vi "SimpleMotorFF_MinAchieveVel.vi"(9 "Acceleration":dbl, 10 "MaxVoltage":dbl, 11 "SIMPLE_MOTOR_FF":T1 {"Ka" format="%13.4f"; "Kv" format="%13.4f"; "Ks" format="%13.4f"}) -> (3 "MinVelocity":dbl)   [LabVIEW 2019, in "Trajectory_Library.lvlib"]
doc: "Calculates the minimum achievable velocity given a maximum voltage supply and an acceleration. Useful for ensuring that velocity and acceleration constraints for a trapezoidal profile are simultaneously achievable - enter the acceleration constraint, and this will give you a simultaneously-achievable velocity constraint.\n\nParameters:\n - Simple_Motor_FF - Data structure containing constants\n - maxVoltage -The maximum voltage that can be supplied to the motor.\n - Acceleration - The acceleration of the motor.\n\nReturns:\n - MinVelocity - The minimum possible velocity at the given acceleration."
uses:
  Trajectory_Library.lvlib
  TypeDef/SIMPLE_MOTOR_FF.ctl
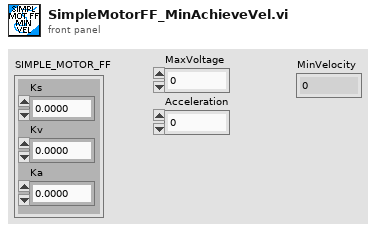
[diagram p1: front panel]
types:
  T1 = typedef "Trajectory_Library.lvlib/SIMPLE_MOTOR_FF.ctl" = cluster{"Ks":dbl, "Kv":dbl, "Ka":dbl}
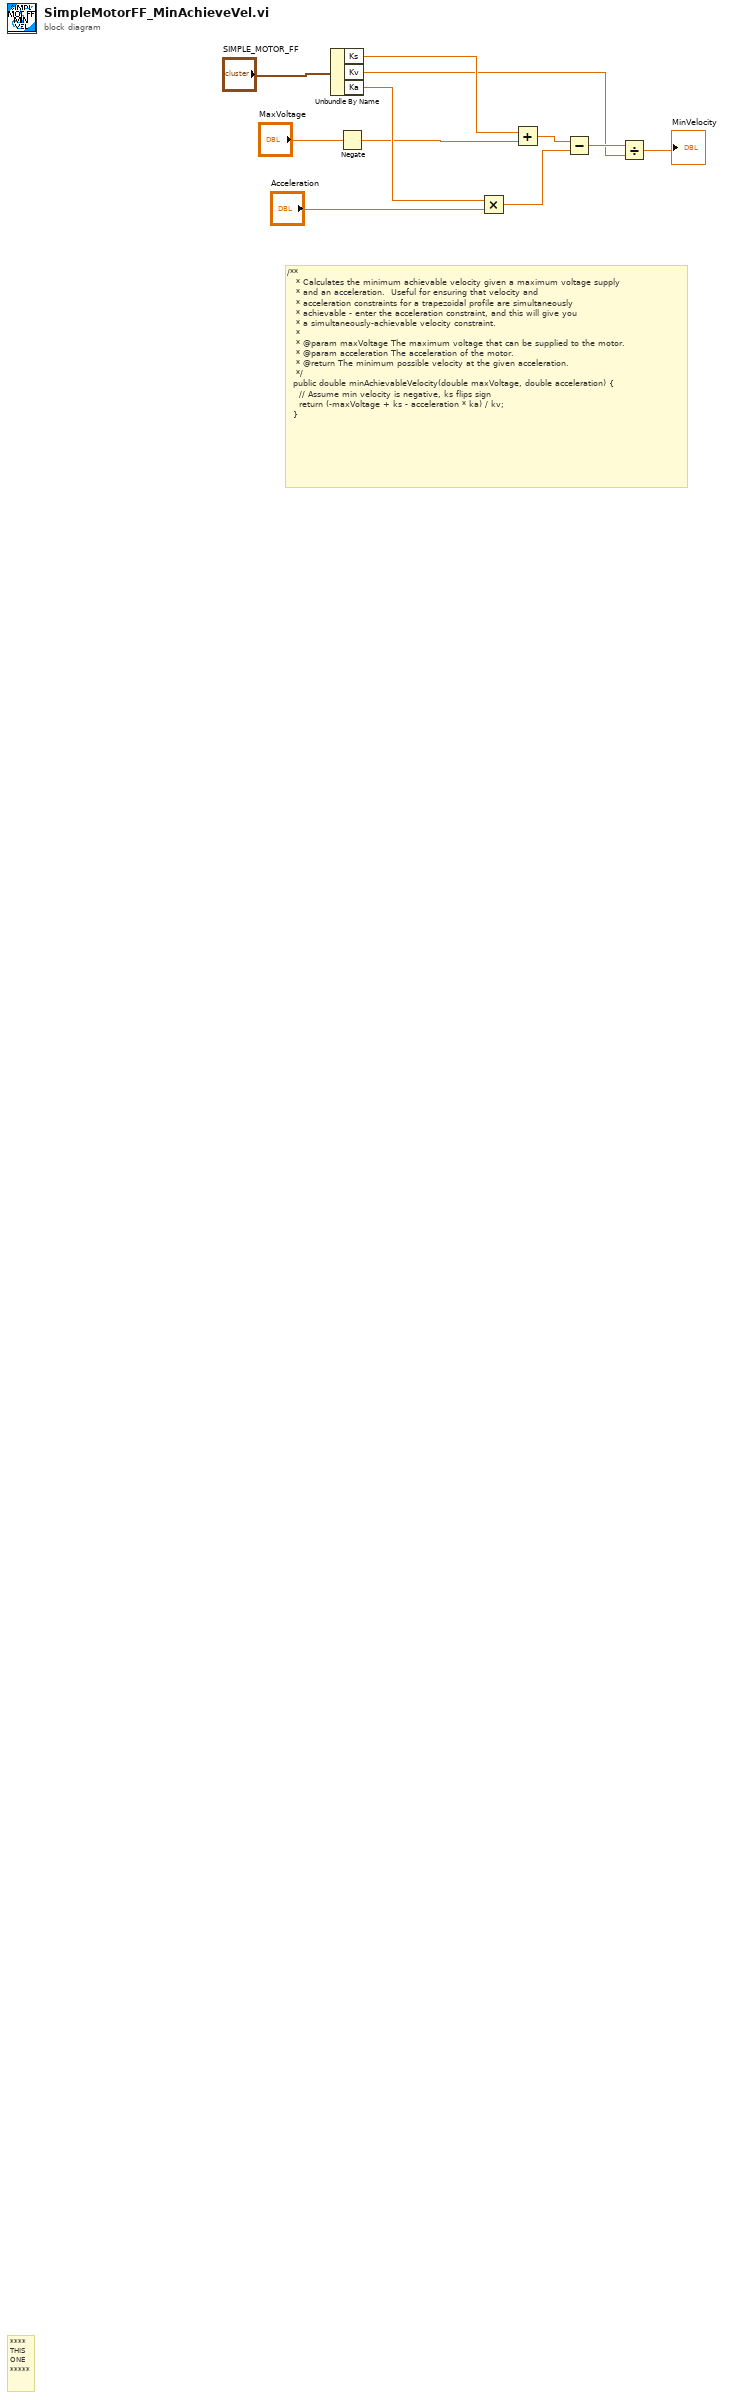
[diagram p0: block diagram]
diagram:
  # "/**\n   * Calculates the minimum achievable velocity given a maximum voltage supply\n   * and an acceleration.  Useful for ensuring that velocity and\n   * acceleration constraints for a trapezoidal profile are simultaneously\n   * achievable - enter the acceleration constraint, and this will give you\n   * a simultaneously-achievable velocity constraint.\n   *\n   * @param maxVoltage The maximum voltage that can be supplied to the motor.\n   * @param acceleration The acceleration of the motor.\n   * @return The minimum possible velocity at the given acceleration.\n   */\n  public double minAchievableVelocity(double maxVoltage, double acceleration) {\n    // Assume min velocity is negative, ks flips sign\n    return (-maxVoltage + ks - acceleration * ka) / kv;\n  }"
  # "****\nTHIS\nONE\n*****"
  n1 = Unbundle By Name("SIMPLE_MOTOR_FF") -> ("Ks"=w9:dbl, "Kv"=w7:dbl, "Ka"=w8:dbl)
  n2 = Negate(x="MaxVoltage") -> (-x=w5:dbl)
  n3 = Multiply(x=w8, y="Acceleration") -> (x*y=w2:dbl)
  n4 = Add(x=w9, y=w5) -> (x+y=w4:dbl)
  n5 = Subtract(x=w4, y=w2) -> (x-y=w10:dbl)
  n6 = Divide(x=w10, y=w7) -> (x/y=→"MinVelocity":dbl)
